vi "Magnetic Field.vi"(8 "error in (no error)":errorcluster, 10 "Power Supply in":refnum<class "Power Supply.lvclass">, 11 "Magnetic Field.lvclass in":refnum<class "Magnetic Field.lvclass">) -> (0 "error out":errorcluster, 3 "Magnetic Field.lvclass out":refnum<class "Magnetic Field.lvclass">)   [LabVIEW 2009, in "Magnetic Field.lvclass"]
uses:
  Magnetic Field.lvclass
  Instruments/Magnet/Power Supply/Power Supply.lvclass
  Scanner/Scanner.lvclass
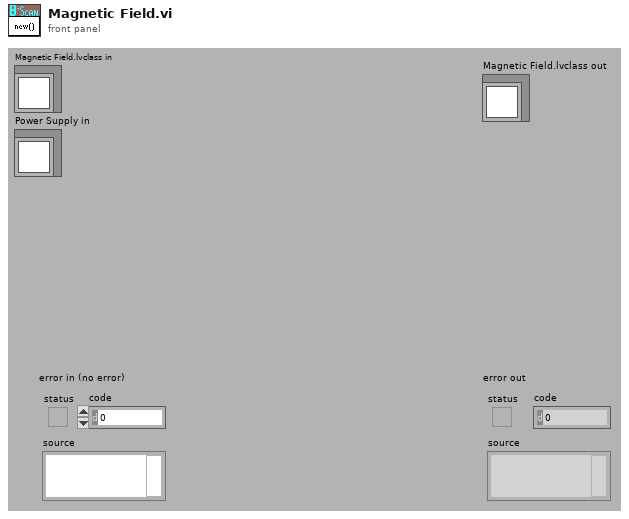
[diagram p1: front panel]
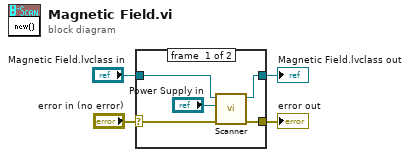
[diagram p0: block diagram]
diagram:
  n1 = case shown="No Error" "error in (no error)" {
    selector: "error in (no error)" -> [w9 w10]
    tunnel: [w8 w10] -> w3
    tunnel: [w6 w11] -> w1
    tunnel: "Magnetic Field.lvclass in" -> [w7 w11]
    frame #0 {
      n2 = call "Scanner.vi"("error in (no error)"=w9, "Scannable"="Power Supply in", "Scanner.lvclass in"=w7) -> ("error out"=w8:errorcluster, "Scanner.lvclass out"=w6:refnum<class "Magnetic Field.lvclass">)  [unwired: 1 in, 6 out]
    }
    frame #1 {
    }
  }
  "error out" <- w3
  "Magnetic Field.lvclass out" <- w1
